vi "Login.vi"(4 "error in (no error)":errorcluster, 6 "Password":string, 7 "Login":string) -> (0 "error out":errorcluster, 2 "Access":bool=TRUE, 3 "User":string)   [LabVIEW 2021]
panel:
  in  "Table":string[][](array[string])=[["admin", "labview"], ["user 1", "12345"], ["guest", ""]]
  in  "OK Button":bool
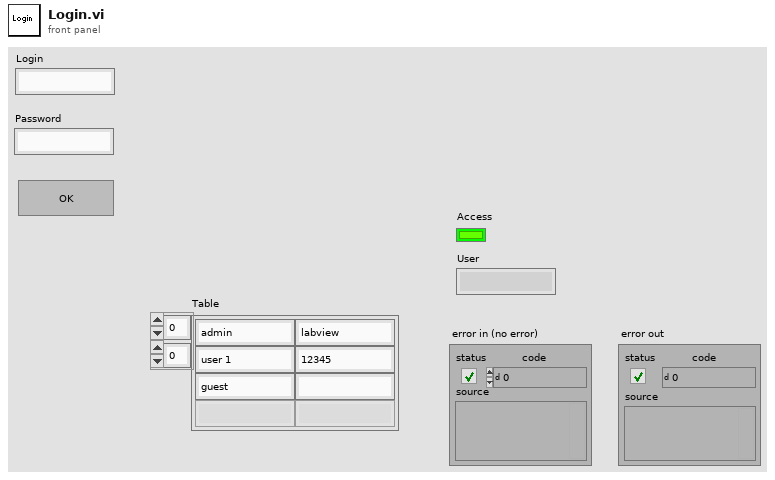
[diagram p1: front panel]
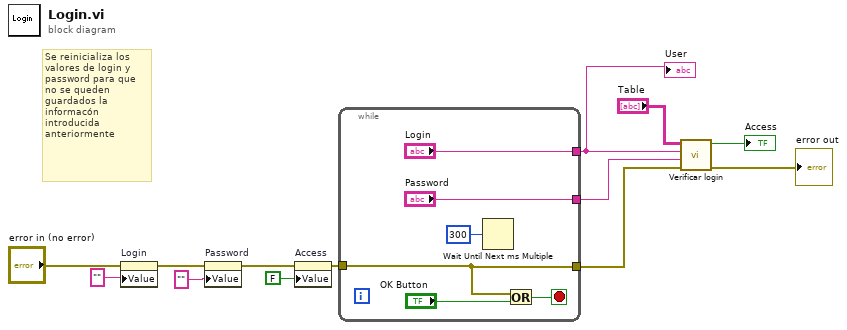
[diagram p0: block diagram]
diagram:
  # "Se reinicializa los valores de login y password para que  no se queden guardados la informacón introducida anteriormente"
  n1 = property on="Login" class="Str"(error in="error in (no error)", "Value"="") -> (error out=w5:errorcluster)  [unwired: 1 in, 1 out]
  n2 = property on="Password" class="Str"(error in=w5, "Value"="" ("Password")) -> (error out=w4:errorcluster)  [unwired: 1 in, 1 out]
  n3 = property on="Access" class="Bool (strict)"(error in=w4, "Value"=FALSE) -> (error out=w3:errorcluster)  [unwired: 1 in, 1 out]
  n4 = while {
    tunnel: ["Password"] -> w8
    tunnel: ["Login"] -> w9
    tunnel: w3 -> [w14]
    tunnel: [w14] -> w2
    stop <- w15 stop-if-true
    n5 = Wait Until Next ms Multiple(millisecond multiple=u32 300) -> ()  [unwired: 1 out]
    n6 = Or(x=w14, y="OK Button") -> (x .or. y?=w15:bool)
  }
  "User" <- w9
  n7 = call "Verificar login.vi"("error in (no error)"=w2, "Password"=w8, "Login"=w9, "Table"="Table") -> ("error out"=→"error out":errorcluster, "Verificado"=→"Access":bool)  [unwired: 2 in]
